vi "__MPI_move_pos_RS232c.vi"(4 "pos":dbl=10.0 format="%#.5g", 7 "VISAリソース名":refnum<visa-resource-name>="COM5") -> (3 "®ì»ÝÊu":string="10.00000\r\n")   [LabVIEW 2017]
uses:
  <vilib>/Instr/_visa.llb/VISA Configure Serial Port (Instr).vi
panel:
  in  "wait":i32=10
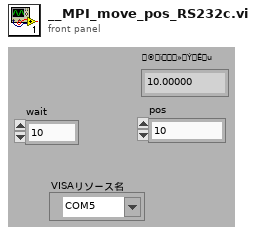
[diagram p1: front panel]
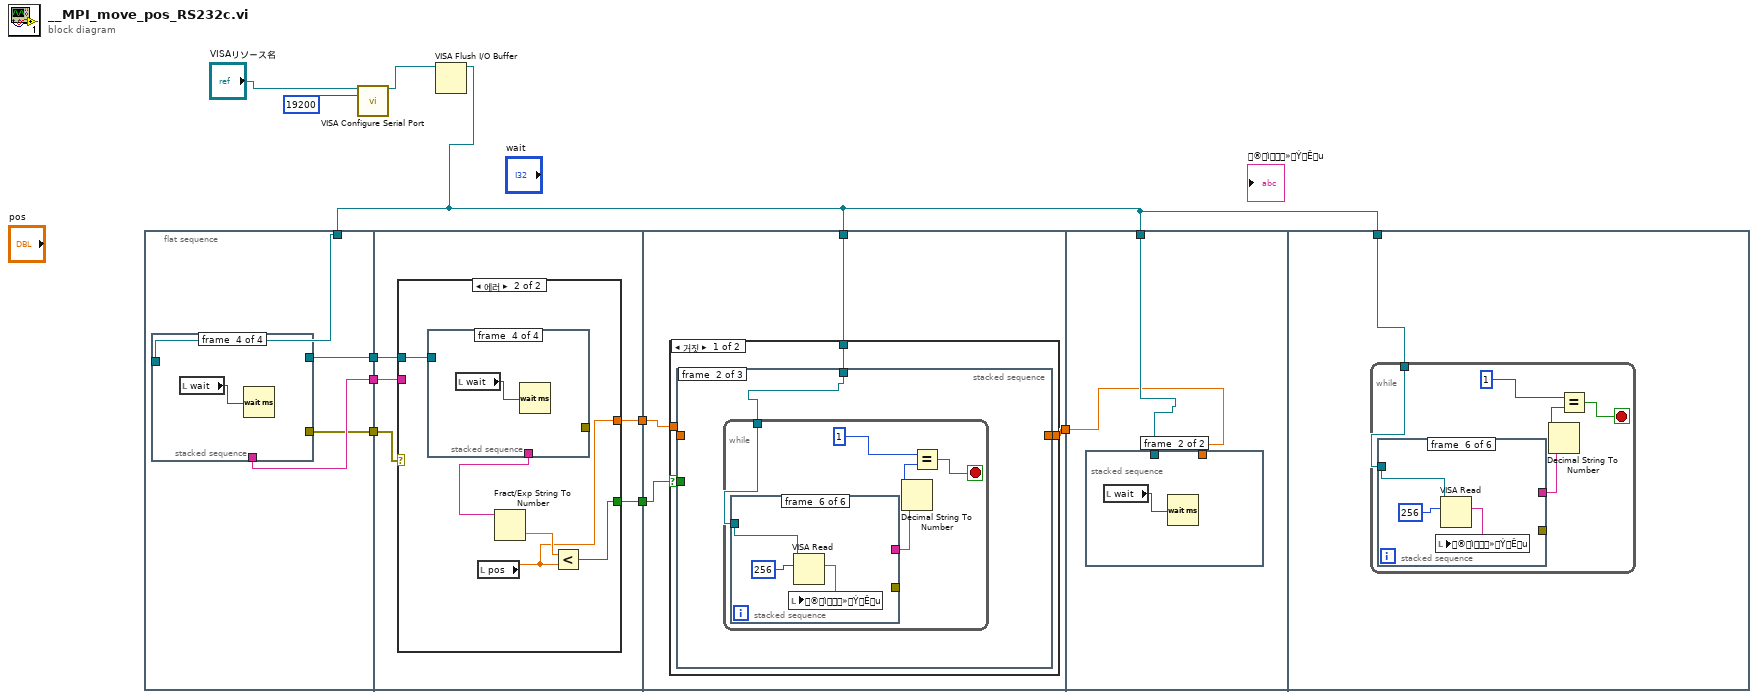
[diagram p0: block diagram]
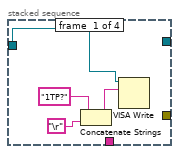
[diagram p2: hidden frame]
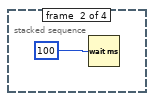
[diagram p3: hidden frame]
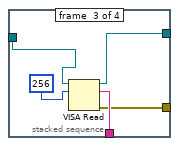
[diagram p4: hidden frame]
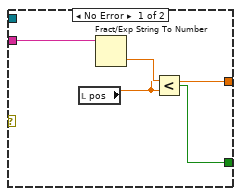
[diagram p5: hidden frame]
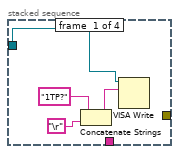
[diagram p6: hidden frame]
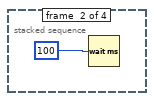
[diagram p7: hidden frame]
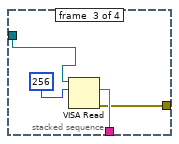
[diagram p8: hidden frame]
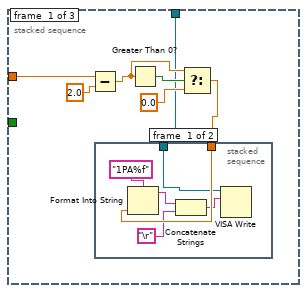
[diagram p9: hidden frame]
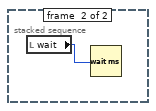
[diagram p10: hidden frame]
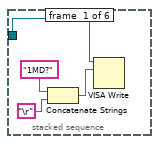
[diagram p11: hidden frame]
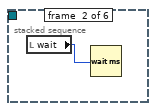
[diagram p12: hidden frame]
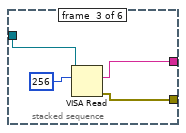
[diagram p13: hidden frame]
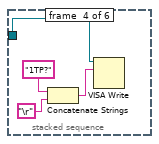
[diagram p14: hidden frame]
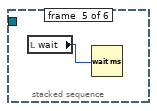
[diagram p15: hidden frame]
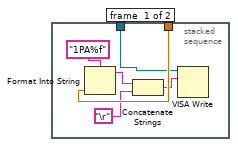
[diagram p18: hidden frame]
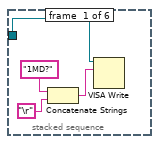
[diagram p19: hidden frame]
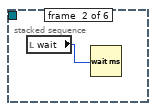
[diagram p20: hidden frame]
diagram:
  n1 = flat-sequence {
    tunnel: w6 -> [w14]
    tunnel: [w13] -> w3
    tunnel: [w12] -> w2
    tunnel: [w11] -> w1
    tunnel: [w29] -> w5
    tunnel: [w30] -> w4
    tunnel: w3 -> [w28]
    tunnel: w2 -> [w27]
    tunnel: w1 -> [w26]
    tunnel: w5 -> [w53]
    tunnel: w4 -> [w52]
    tunnel: w6 -> [w51]
    tunnel: [w50] -> w10
    tunnel: w6 -> [w98]
    tunnel: w10 -> [w97]
    tunnel: w6 -> [w106]
    frame #0 {
      n2 = stacked-sequence {
        tunnel: w14 -> [w18 _ w24 _]
        tunnel: [_ _ w23 _] -> w13
        tunnel: [_ _ w21 _] -> w12
        tunnel: [_ _ w20 _] -> w11
        frame #0 {
          n3 = Concatenate Strings("1TP?", "\r") -> (w15:string)
          n4 = VISA Write(VISA resource name=w18, write buffer=w15) -> ()  [unwired: 1 in, 3 out]
        }
        frame #1 {
          n5 = Wait (ms)(milliseconds to wait=100) -> ()  [unwired: 1 out]
        }
        frame #2 {
          n6 = VISA Read(VISA resource name=w24, byte count=256) -> (VISA resource name out=w20:refnum<visa-resource-name>, read buffer=w23:string, error out=w21:errorcluster)  [unwired: 1 in, 1 out]
        }
        frame #3 {
          n7 = local read "wait"() -> (w25:i32)
          n8 = Wait (ms)(milliseconds to wait=w25) -> ()  [unwired: 1 out]
        }
      }
    }
    frame #1 {
      n9 = case shown="에러" w27 {
        tunnel: [w31 w35] -> w30
        tunnel: [w33 w36] -> w29
        tunnel: w28 -> [w32 _]
        tunnel: w26 -> [_ w39]
        frame No Error {
          n10 = local read "pos"() -> (w31:dbl)
          n11 = Fract/Exp String To Number(string=w32) -> (number=w34:dbl)  [unwired: 3 in, 1 out]
          n12 = Less?(x=w34, y=w31) -> (x < y?=w33:bool)
        }
        frame Error {
          n13 = stacked-sequence {
            tunnel: w39 -> [w43 _ w48 _]
            tunnel: [_ _ w47 _] -> w37
            tunnel: [_ _ w45 _] -> _
            frame #0 {
              n14 = Concatenate Strings("1TP?", "\r") -> (w40:string)
              n15 = VISA Write(VISA resource name=w43, write buffer=w40) -> ()  [unwired: 1 in, 3 out]
            }
            frame #1 {
              n16 = Wait (ms)(milliseconds to wait=100) -> ()  [unwired: 1 out]
            }
            frame #2 {
              n17 = VISA Read(VISA resource name=w48, byte count=256) -> (read buffer=w47:string, error out=w45:errorcluster)  [unwired: 1 in, 2 out]
            }
            frame #3 {
              n18 = local read "wait"() -> (w49:i32)
              n19 = Wait (ms)(milliseconds to wait=w49) -> ()  [unwired: 1 out]
            }
          }
          n20 = local read "pos"() -> (w35:dbl)
          n21 = Fract/Exp String To Number(string=w37) -> (number=w38:dbl)  [unwired: 3 in, 1 out]
          n22 = Less?(x=w38, y=w35) -> (x < y?=w36:bool)
        }
      }
    }
    frame #2 {
      n23 = case shown="거짓" w53 {
        selector: w53 -> [w54 _]
        tunnel: w52 -> [w57 w96]
        tunnel: w51 -> [w56 _]
        tunnel: [w55 w96] -> w50
        frame False {
          n24 = stacked-sequence {
            tunnel: w57 -> [w60 _ w95]
            tunnel: w56 -> [w59 w72 _]
            tunnel: [_ _ w95] -> w55
            tunnel: w54 -> [_ _ _]
            frame #0 {
              n25 = Subtract(x=w60, y=2.0) -> (x-y=w62:dbl)
              n26 = Greater Than 0?(x=w62) -> (x > 0?=w63:bool)
              n27 = Select(t=w62, s=w63, f=0.0) -> (s? t:f=w58:dbl)
              n28 = stacked-sequence {
                tunnel: w59 -> [w68 _]
                tunnel: w58 -> [w69 _]
                frame #0 {
                  n29 = Format Into String(format string="1PA%f", w69) -> (resulting string=w67:string)  [unwired: 2 in, 1 out]
                  n30 = Concatenate Strings(w67, "\r") -> (w66:string)
                  n31 = VISA Write(VISA resource name=w68, write buffer=w66) -> ()  [unwired: 1 in, 3 out]
                }
                frame #1 {
                  n32 = local read "wait"() -> (w71:i32)
                  n33 = Wait (ms)(milliseconds to wait=w71) -> ()  [unwired: 1 out]
                }
              }
            }
            frame #1 {
              n34 = while {
                tunnel: w72 -> [w73]
                stop <- w76 stop-if-true
                n35 = stacked-sequence {
                  tunnel: w73 -> [w81 _ w85 w90 _ w93]
                  tunnel: [_ _ w83 _ _ _] -> w74
                  tunnel: [_ _ w84 _ _ _] -> _
                  frame #0 {
                    n36 = Concatenate Strings("1MD?", "\r") -> (w78:string)
                    n37 = VISA Write(VISA resource name=w81, write buffer=w78) -> ()  [unwired: 1 in, 3 out]
                  }
                  frame #1 {
                    n38 = local read "wait"() -> (w82:i32)
                    n39 = Wait (ms)(milliseconds to wait=w82) -> ()  [unwired: 1 out]
                  }
                  frame #2 {
                    n40 = VISA Read(VISA resource name=w85, byte count=256) -> (read buffer=w83:string, error out=w84:errorcluster)  [unwired: 1 in, 2 out]
                  }
                  frame #3 {
                    n41 = Concatenate Strings("1TP?", "\r") -> (w87:string)
                    n42 = VISA Write(VISA resource name=w90, write buffer=w87) -> ()  [unwired: 1 in, 3 out]
                  }
                  frame #4 {
                    n43 = local read "wait"() -> (w91:i32)
                    n44 = Wait (ms)(milliseconds to wait=w91) -> ()  [unwired: 1 out]
                  }
                  frame #5 {
                    n45 = VISA Read(VISA resource name=w93, byte count=256) -> (read buffer=w92:string)  [unwired: 1 in, 3 out]
                    n46 = local write "®ì»ÝÊu"(w92) -> ()
                  }
                }
                n47 = Decimal String To Number(string=w74) -> (number=w75:i32)  [unwired: 2 in, 1 out]
                n48 = Equal?(x=1, y=w75) -> (x = y?=w76:bool)
              }
            }
            frame #2 {
            }
          }
        }
        frame True {
        }
      }
    }
    frame #3 {
      n49 = stacked-sequence {
        tunnel: w98 -> [w102 _]
        tunnel: w97 -> [w103 _]
        frame #0 {
          n50 = Format Into String(format string="1PA%f", w103) -> (resulting string=w101:string)  [unwired: 2 in, 1 out]
          n51 = Concatenate Strings(w101, "\r") -> (w100:string)
          n52 = VISA Write(VISA resource name=w102, write buffer=w100) -> ()  [unwired: 1 in, 3 out]
        }
        frame #1 {
          n53 = local read "wait"() -> (w105:i32)
          n54 = Wait (ms)(milliseconds to wait=w105) -> ()  [unwired: 1 out]
        }
      }
    }
    frame #4 {
      n55 = while {
        tunnel: w106 -> [w107]
        stop <- w110 stop-if-true
        n56 = stacked-sequence {
          tunnel: w107 -> [w115 _ w119 w124 _ w127]
          tunnel: [_ _ w117 _ _ _] -> w108
          tunnel: [_ _ w118 _ _ _] -> _
          frame #0 {
            n57 = Concatenate Strings("1MD?", "\r") -> (w112:string)
            n58 = VISA Write(VISA resource name=w115, write buffer=w112) -> ()  [unwired: 1 in, 3 out]
          }
          frame #1 {
            n59 = local read "wait"() -> (w116:i32)
            n60 = Wait (ms)(milliseconds to wait=w116) -> ()  [unwired: 1 out]
          }
          frame #2 {
            n61 = VISA Read(VISA resource name=w119, byte count=256) -> (read buffer=w117:string, error out=w118:errorcluster)  [unwired: 1 in, 2 out]
          }
          frame #3 {
            n62 = Concatenate Strings("1TP?", "\r") -> (w121:string)
            n63 = VISA Write(VISA resource name=w124, write buffer=w121) -> ()  [unwired: 1 in, 3 out]
          }
          frame #4 {
            n64 = local read "wait"() -> (w125:i32)
            n65 = Wait (ms)(milliseconds to wait=w125) -> ()  [unwired: 1 out]
          }
          frame #5 {
            n66 = VISA Read(VISA resource name=w127, byte count=256) -> (read buffer=w126:string)  [unwired: 1 in, 3 out]
            n67 = local write "®ì»ÝÊu"(w126) -> ()
          }
        }
        n68 = Decimal String To Number(string=w108) -> (number=w109:i32)  [unwired: 2 in, 1 out]
        n69 = Equal?(x=1, y=w109) -> (x = y?=w110:bool)
      }
    }
  }
  n70 = call-poly "VISA Configure Serial Port"("VISA resource name"="VISAリソース名", "baud rate (9600)"=19200) -> ("VISA resource name out"=w7:refnum<visa-resource-name>)  [unwired: 12 in, 1 out]
  n71 = VISA Flush I/O Buffer(VISA resource name=w7) -> (VISA resource name out=w6:refnum<visa-resource-name>)  [unwired: 2 in, 1 out]
